vi "Reset Display.vi"(6 "Array":refnum<vi>[](array[refnum]), 8 "error in (no error)":errorcluster, 9 "Boolean":refnum<vi>, 10 "Result Graph":refnum<vi>, 11 "Tab Control":refnum<vi>) -> (0 "error out":errorcluster)   [LabVIEW 2017]
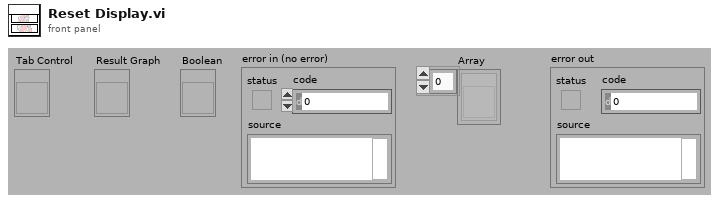
[diagram p1: front panel]
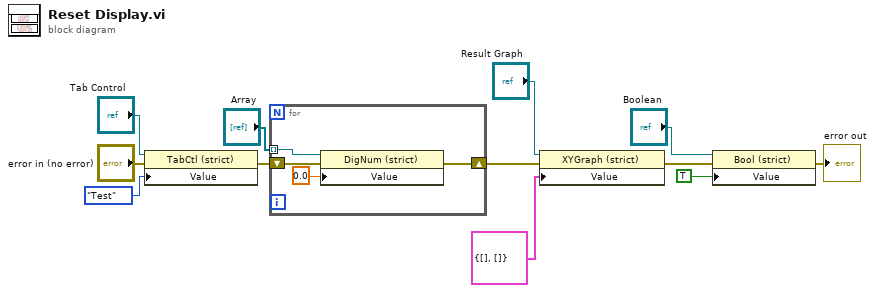
[diagram p0: block diagram]
diagram:
  n1 = property class="TabCtl (strict)"(reference="Tab Control", error in="error in (no error)", "Value"=enum32{"Test", "Results"}."Test") -> (error out=w12:errorcluster)  [unwired: 1 out]
  n2 = for {
    tunnel: "Array" -> [w14] mode=indexing
    shift-right: [w15] -> w4
    shift-left: w12 -> [w13]
    n3 = property class="DigNum (strict)"(reference=w14, error in=w13, "Value"=0.0) -> (error out=w15:errorcluster)  [unwired: 1 out]
  }
  n4 = property class="XYGraph (strict)"(reference="Result Graph", error in=w4, "Value"=cluster{dbl[], dbl[]} {[], []}) -> (error out=w1:errorcluster)  [unwired: 1 out]
  n5 = property class="Bool (strict)"(reference="Boolean", error in=w1, "Value"=TRUE) -> (error out=→"error out":errorcluster)  [unwired: 1 out]
